vi "Bank Shot.vi"(8 "L (ft)":dbl=12.0, 9 "Camera (deg)":dbl, 10 "Turret (deg)":dbl=-180.0, 11 "Gryo (deg)":dbl) -> (0 "Distance from center (in)":dbl, 3 "C Prime":dbl)   [LabVIEW 2013]
panel:
  out "Theta Prime (or B)":dbl
  out "Theta":dbl
  out "B (deg)":dbl
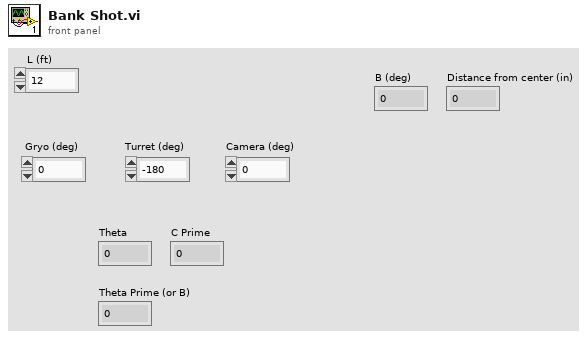
[diagram p1: front panel]
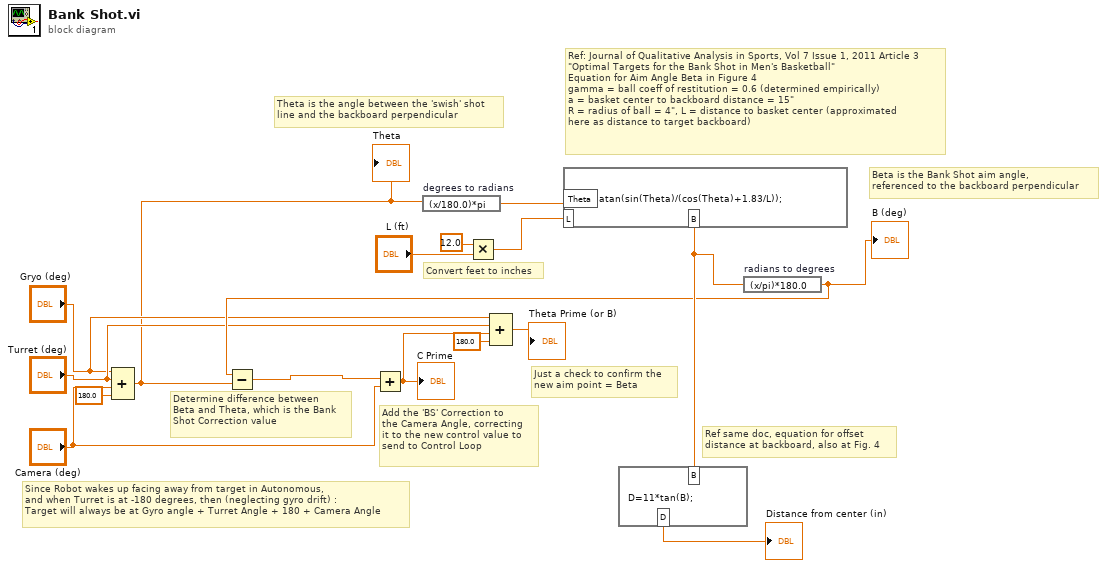
[diagram p0: block diagram]
diagram:
  # "Convert feet to inches"
  # "Beta is the Bank Shot aim angle, \nreferenced to the backboard perpendicular"
  # "Theta is the angle between the 'swish' shot\nline and the backboard perpendicular"
  # "Since Robot wakes up facing away from target in Autonomous,\nand when Turret is at -180 degrees, then (neglecting gyro drift) :\nTarget will always be at Gyro angle + Turret Angle + 180 + Camera Angle"
  # "Ref same doc, equation for offset\ndistance at backboard, also at Fig. 4"
  # "Ref: Journal of Qualitative Analysis in Sports, Vol 7 Issue 1, 2011 Article 3\n\"Optimal Targets for the Bank Shot in Men's Basketball\"\nEquation for Aim Angle Beta in Figure 4\ngamma = ball coeff of restitution = 0.6 (determined empirically)\na = basket center to backboard distance = 15\"\nR = radius of ball = 4\", L = distance to basket center (approximated \nhere as distance to target backboard)"
  # "Just a check to confirm the\nnew aim point = Beta"
  # "Add the 'BS' Correction to\nthe Camera Angle, correcting\nit to the new control value to \nsend to Control Loop"
  # "Determine difference between\nBeta and Theta, which is the Bank\nShot Correction value"
  n1 = Compound Arithmetic op=ADD("Gryo (deg)", "Turret (deg)", "Camera (deg)", 180.0 ("value")) -> (w2:dbl)
  "Theta" <- w2
  n2 = expression code="(x/180.0)*pi" "degrees to radians"(w2) -> (w13:dbl)
  n3 = Multiply(x=12.0, y="L (ft)") -> (x*y=w15:dbl)
  n4 = formula code="B  =  atan(sin(Theta)/(cos(Theta)+1.83/L));"("Theta"=w13, "L"=w15) -> ("B"=w11:dbl)
  n5 = formula code="D=11*tan(B);"("B"=w11) -> ("D"=→"Distance from center (in)":dbl)
  n6 = expression code="(x/pi)*180.0" "radians to degrees"(w11) -> (w9:dbl)
  "B (deg)" <- w9
  n7 = Subtract(x=w9, y=w2) -> (x-y=w1:dbl)
  n8 = Add(x=w1, y="Camera (deg)") -> (x+y=w8:dbl)
  "C Prime" <- w8
  n9 = Compound Arithmetic op=ADD("Gryo (deg)", "Turret (deg)", w8, 180.0 ("value")) -> (→"Theta Prime (or B)":dbl)
